vi "Open.vi"(8 "error in (no error)":errorcluster, 11 "Serial Port":string) -> (0 "error out":errorcluster, 3 "FW102C out":i32, 5 "Connected?":bool)   [LabVIEW 2017, in "Colour Wheel.lvlib" / "Thorlabs_FW102C.lvlib"]
uses:
  Thorlabs_FW102C.lvlib
  <vilib>/Utility/error.llb/Error Cluster From Error Code.vi
  <vilib>/ErrorRing/Error Ring.xnode
  Library/FilterWheel102_win32.dll
  Library/FilterWheel102_win64.dll
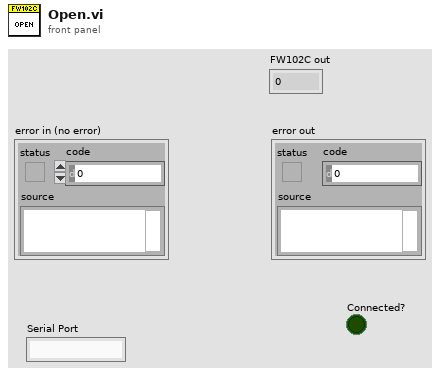
[diagram p1: front panel]
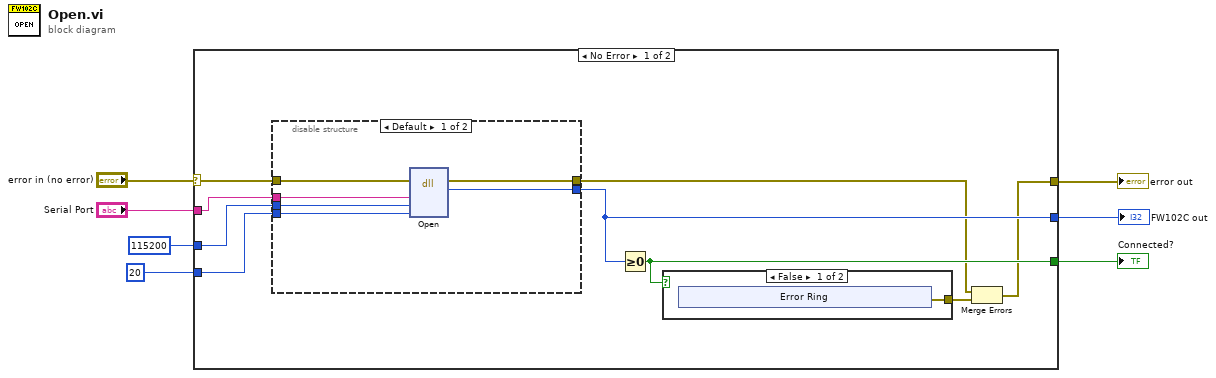
[diagram p0: block diagram]
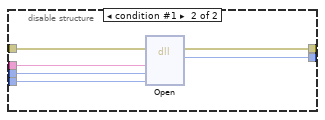
[diagram p3: hidden frame]
diagram:
  n1 = case shown="No Error" "error in (no error)" {
    selector: "error in (no error)" -> [w16 w35]
    tunnel: [w8 w35] -> w6
    tunnel: 20 ("timeout") -> [w14 _]
    tunnel: "Serial Port" -> [w15 _]
    tunnel: [w11 _] -> w3
    tunnel: [w12 _] -> w2
    tunnel: 115200 ("nbaud") -> [w13 _]
    frame No Error {
      n2 = disable-structure shown="Default" {
        disable-tunnel: w16 -> [w28 w34]
        disable-tunnel: [w27 w33] -> w9
        disable-tunnel: w15 -> [w26 w32]
        disable-tunnel: w14 -> [w25 w31]
        disable-tunnel: w13 -> [w24 w30]
        disable-tunnel: [w23 w29] -> w12
        frame condition #0 (active) {
          n3 = dll-call lib="C:/Project Work/icl-optical-software-rewrite/Optical Software Code Simplified/Modules/Colour Wheel/Thorlabs_FW102C/Library/FilterWheel102_win32.dll" fn="Open"(error in=w28, "Serial No"=w26, "nBaud"=w24, "timeout"=w25) -> (error out=w27:errorcluster, "hdl"=w23:i32)  [unwired: 5 in, 1 out]
        }
        frame condition #1 {
          n4 = dll-call lib="C:/Project Work/icl-optical-software-rewrite/Optical Software Code Simplified/Modules/Colour Wheel/Thorlabs_FW102C/Library/FilterWheel102_win64.dll" fn="Open"(error in=w34, "Serial No"=w32, "nBaud"=w30, "timeout"=w31) -> (error out=w33:errorcluster, "hdl"=w29:i32)  [unwired: 5 in, 1 out]
        }
      }
      n5 = Greater Or Equal To 0?(x=w12) -> (x >= 0?=w11:bool)
      n6 = case shown="False" w11 {
        tunnel: [w17 _] -> w10
        frame False {
          n7 = xnode "Error Ring"() -> ("error out"=w17:errorcluster)
        }
        frame True {
        }
      }
      n8 = Merge Errors(w9, w10) -> (w8:errorcluster)
    }
    frame Error {
    }
  }
  "error out" <- w6
  "Connected?" <- w3
  "FW102C out" <- w2
